vi "配置写入.vi"(8 "error in (no error)":errorcluster caption="错误输入（无错误）", 11 "数据值":T1) -> (0 "error out":errorcluster caption="错误输出")   [LabVIEW 2016, in "TimingControl.lvlib" / "TimingControl.lvclass"]
uses:
  TimingControl.lvclass
  State Data.ctl
  <vilib>/Utility/xml.llb/Write to XML File(string).vi
panel:
  # "分钟"
  # "次"
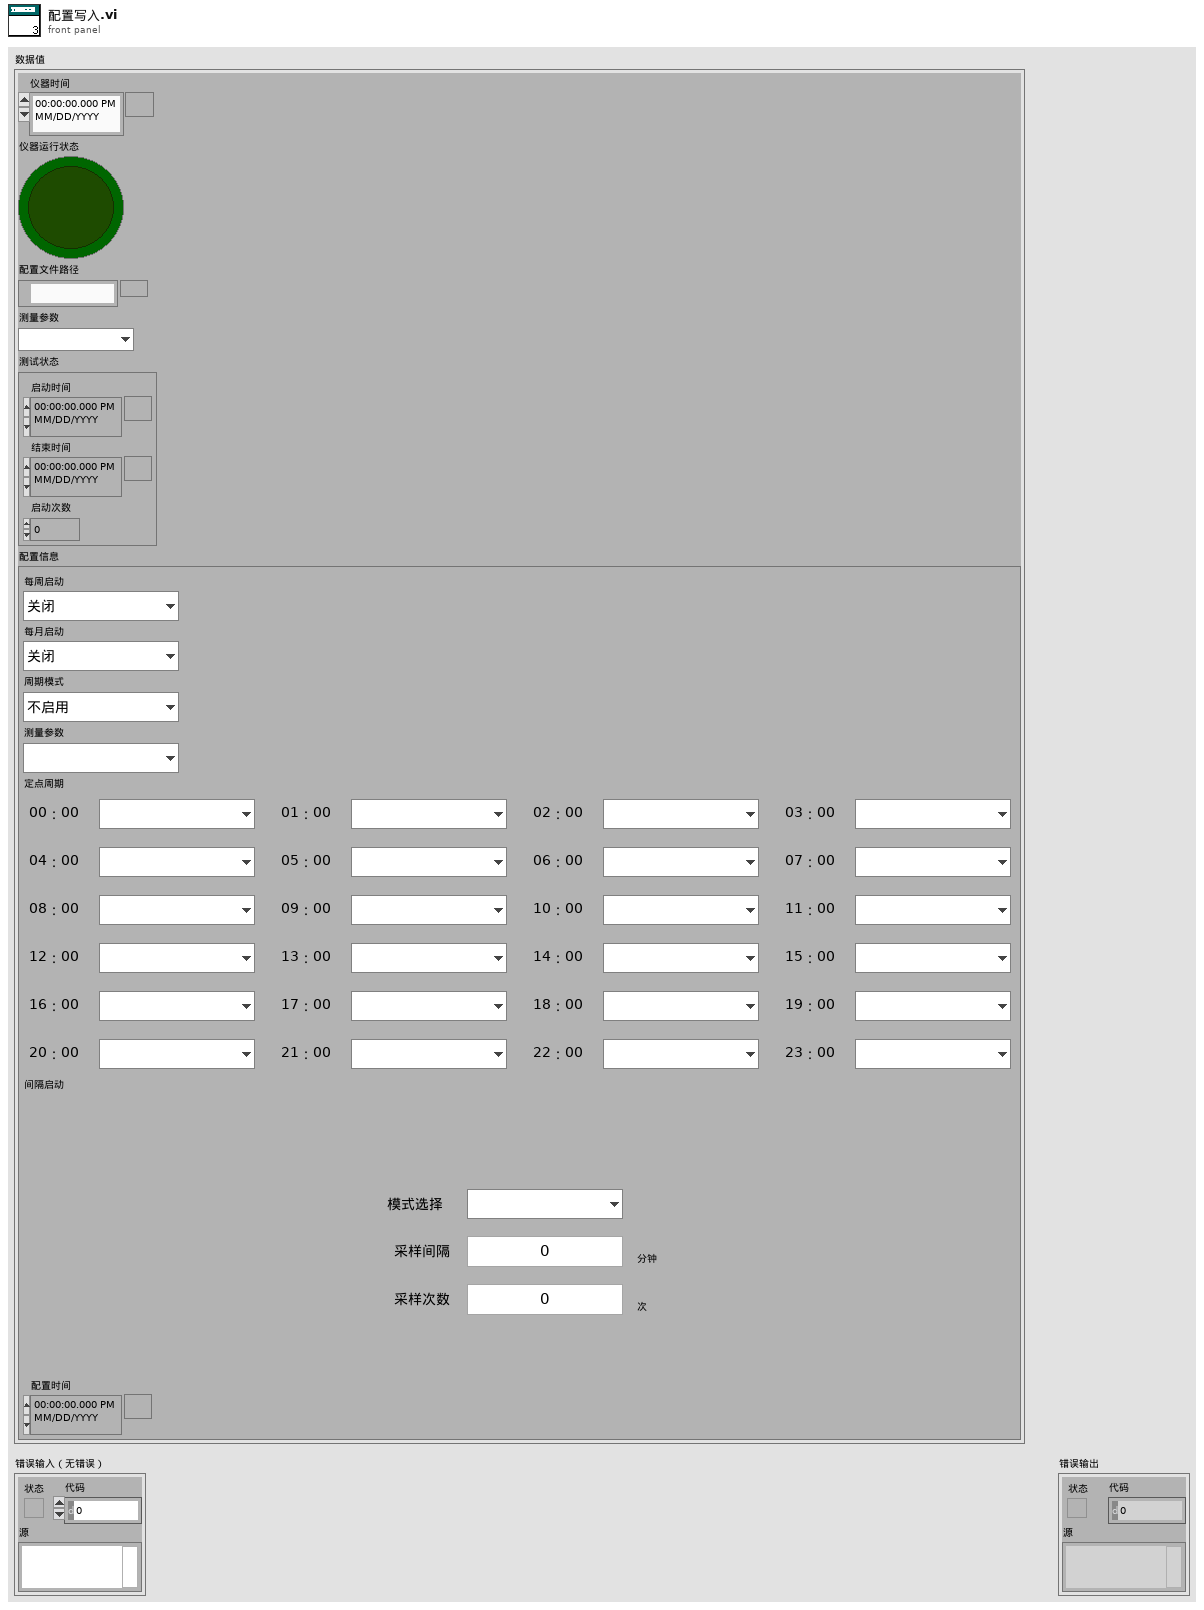
[diagram p1: front panel]
types:
  T1 = typedef "TimingControl.lvlib/TimingControl.lvclass/State Data.ctl" = cluster{"仪器时间":timestamp, "仪器运行状态":bool, "配置文件路径":path, "测量参数":u16, "测试状态":cluster{"启动时间":timestamp, "结束时间":timestamp, "启动次数":i32}, "配置信息":T2}
  T2 = typedef "TimingControl.lvlib/TimingControl.lvclass/配置信息.ctl" = cluster{"每周启动":T3, "每月启动":T4, "周期模式":T5, "测量参数":T6, "定点周期":T7, "间隔启动":T9, "配置时间":timestamp}
  T3 = typedef "TimingControl.lvlib/TimingControl.lvclass/每周启动.ctl" = enum16{"关闭", "周日", "周一", "周二", "周三", "周四", "周五", "周六"}
  T4 = typedef "TimingControl.lvlib/TimingControl.lvclass/每月启动.ctl" = enum16{"关闭", "1号", "2号", "3号", "4号", "5号", "6号", "7号", "8号", "9号", "10号", "11号", "12号", "13号", "14号", "15号", "16号", "17号", "18号", "19号", "20号", "21号", "22号", "23号", "24号", "25号", "26号", "27号", "28号", "29号", "30号", "31号"}
  T5 = typedef "TimingControl.lvlib/TimingControl.lvclass/周期模式设置.ctl" = enum16{"不启用", "定点模式", "间隔模式"}
  T6 = typedef "TimingControl.lvlib/TimingControl.lvclass/测量参数.ctl" = u16
  T7 = typedef "TimingControl.lvlib/TimingControl.lvclass/定点周期设置.ctl" = cluster{"启动命令":T8, "启动命令 2":T8, "启动命令 3":T8, "启动命令 4":T8, "启动命令 5":T8, "启动命令 6":T8, "启动命令 7":T8, "启动命令 8":T8, "启动命令 9":T8, "启动命令 10":T8, "启动命令 11":T8, "启动命令 12":T8, "启动命令 13":T8, "启动命令 14":T8, "启动命令 15":T8, "启动命令 16":T8, "启动命令 17":T8, "启动命令 18":T8, "启动命令 19":T8, "启动命令 20":T8, "启动命令 21":T8, "启动命令 22":T8, "启动命令 23":T8, "启动命令 24":T8}
  T8 = typedef "TimingControl.lvlib/TimingControl.lvclass/启动命令选择.ctl" = enum16{"", "水样测试", "标样核查", "零点核查", "跨度核查", "空白测试", "平行样测试", "加标回收", "空白校准", "标样校准", "初始化(清洗)"}
  T9 = typedef "TimingControl.lvlib/TimingControl.lvclass/间隔启动设置.ctl" = cluster{"启动命令":T8, "启动间隔":dbl, "启动次数":i32}
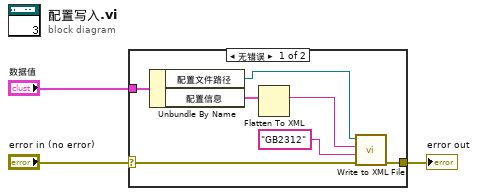
[diagram p0: block diagram]
diagram:
  n1 = case shown="无错误" "error in (no error)" {
    selector: "error in (no error)" -> [w7 w11]
    tunnel: [w6 w11] -> w2
    tunnel: "数据值" -> [w5 _]
    frame No Error {
      n2 = Unbundle By Name(w5) -> ("配置文件路径"=w10:path, "配置信息"=w4:T2)
      n3 = Flatten To XML(anything=w4) -> (xml string=w9:string)
      n4 = call-poly <vilib>:"Write to XML File.vi"("error in (no error)"=w7, "XML Encoding"="GB2312", "XML Input"=w9, "XML File Path"=w10) -> ("error out"=w6:errorcluster)  [unwired: 5 in, 2 out]
    }
    frame Error {
    }
  }
  "error out" <- w2
